vi "AlliGator Build Phasor Ratio Plot Name Prefix.vi"(8 "Error In":errorcluster, 11 "Phasor Plot Name in":string) -> (0 "Error Out":errorcluster, 3 "Phasor Ratio Plot Name Prefix out":string)   [LabVIEW 2021, in "AlliGator Phasor Ratio.lvlib"]
doc: "Strips \" Phasor Plot\" from the source phasor plot name."
uses:
  AlliGator Phasor Ratio.lvlib
panel:
  # "see the AlliGator License on the block diagram (Ctrl+E or Window:Show Block Diagram)"
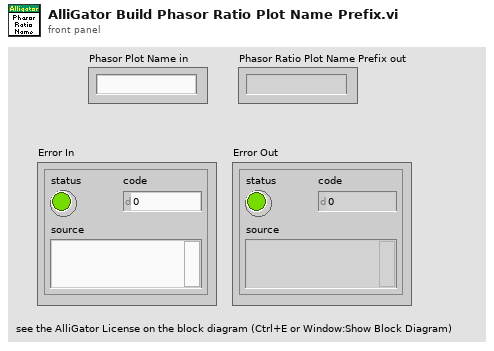
[diagram p1: front panel]
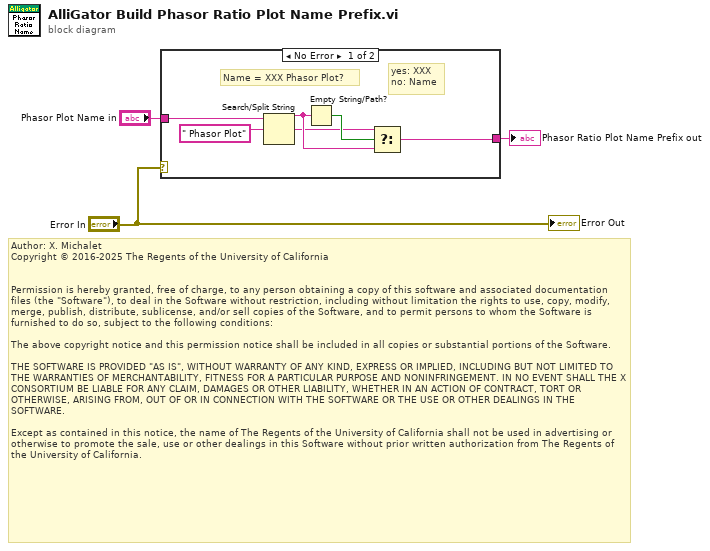
[diagram p0: block diagram]
diagram:
  # "Author: X. Michalet\nCopyright © 2016-2025 The Regents of the University of California\n \n\nPermission is hereby granted, free of charge, to any person obtaining a copy of this software and associated documentation files (the \"Software\"), to deal in the Software without restriction, including without limitation the rights to use, copy, modify, merge, publish, distribute, sublicense, and/or sell copies of the Software, and to permit persons to whom the Software is furnished to do so, subject to the following conditions:\n\nThe above copyright notice and this permission notice shall be included in all copies or substantial portions of the Software.\n\nTHE SOFTWARE IS PROVIDED \"AS IS\", WITHOUT WARRANTY OF ANY KIND, EXPRESS OR IMPLIED, INCLUDING BUT NOT LIMITED TO THE WARRANTIES OF MERCHANTABILITY, FITNESS FOR A PARTICULAR PURPOSE AND NONINFRINGEMENT. IN NO EVENT SHALL THE X CONSORTIUM BE LIABLE FOR ANY CLAIM, DAMAGES OR OTHER LIABILITY, WHETHER IN AN ACTION OF CONTRACT, TORT OR OTHERWISE, ARISING FROM, OUT OF OR IN CONNECTION WITH THE SOFTWARE OR THE USE OR OTHER DEALINGS IN THE SOFTWARE.\n\nExcept as contained in this notice, the name of The Regents of the University of California shall not be used in advertising or otherwise to promote the sale, use or other dealings in this Software without prior written authorization from The Regents of the University of California."
  n1 = case shown="No Error" "Error In" {
    tunnel: [w4 w10] -> w3
    tunnel: "Phasor Plot Name in" -> [w5 w10]
    frame No Error {
      # "yes: XXX\nno: Name"
      # "Name = XXX Phasor Plot?"
      n2 = Search/Split String(string=w5, search string/char (-)=" Phasor Plot") -> (substring before match=w8:string, match + rest of string=w7:string)  [unwired: 1 in, 1 out]
      n3 = Empty String/Path?(string/path=w8) -> (empty?=w9:bool)
      n4 = Select(t=w7, s=w9, f=w8) -> (s? t:f=w4:string)
    }
    frame Error {
    }
  }
  "Phasor Ratio Plot Name Prefix out" <- w3
  "Error Out" <- "Error In"
